vi "SSC DCPower Source Voltage v2.vi"(0 "DCPower SSC in":T1[](array[typedef]), 5 "Voltage Level, V":dbl, 9 "Voltage Level Range (V)":dbl format="%#_6p", 11 "error in":errorcluster, 12 "Current Limit, A":dbl, 14 "Current Limit Range (A)":dbl format="%#_6p") -> (4 "DCPower SSC out":T1[](array[typedef]), 15 "error out":errorcluster)   [LabVIEW 2019]
uses:
  SSC DCPower.ctl
  <instrlib>/niDCPower/nidcpower.llb/niDCPower Output Function.ctl
  <instrlib>/niDCPower/nidcpower.llb/niDCPower Source Mode.ctl
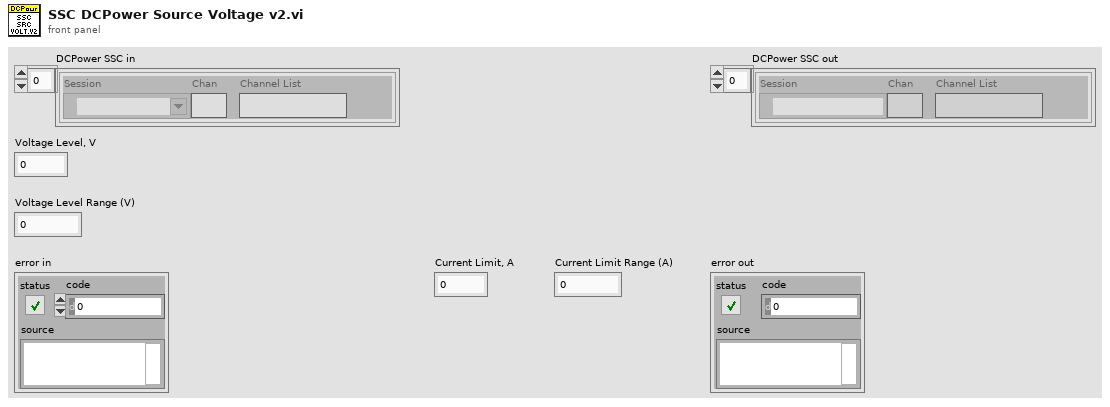
[diagram p1: front panel]
types:
  T1 = typedef "SSC DCPower.ctl" = cluster{"Session":refnum<k15>, "Chan":string, "Channel List":string}
  T2 = typedef "niDCPower Source Mode.ctl" = i32
  T3 = typedef "niDCPower Output Function.ctl" = i32
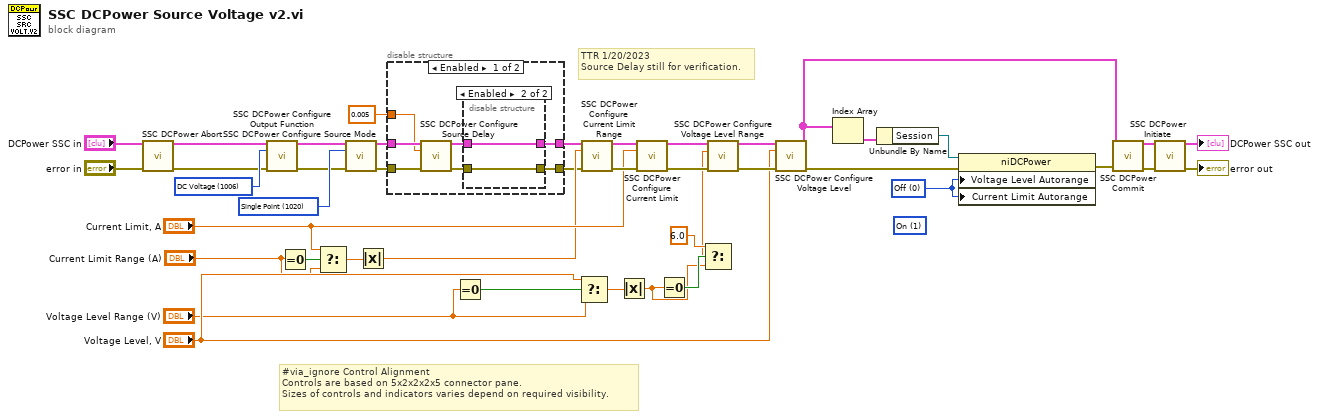
[diagram p0: block diagram]
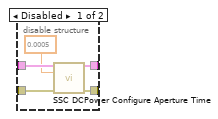
[diagram p2: hidden frame]
diagram:
  (unwired) 1 items=["Off", "On"] ("Source:DC Voltage:Voltage Level Autorange")
  w1 = 0 items=["Off", "On"] ("Source:DC Voltage:Voltage Level Autorange")
  w18 = T2 1020 items=["Single Point"=1020, "Sequence"=1021] ("Source Mode")
  w42 = T3 1006 items=["DC Voltage"=1006, "DC Current"=1007, "Pulse Voltage"=1049, "Pulse Current"=1050] ("Output Function")
  # "TTR 1/20/2023\nSource Delay still for verification."
  # "#via_ignore Control Alignment\nControls are based on 5x2x2x2x5 connector pane.\nSizes of controls and indicators varies depend on required visibility."
  n1 = call "SSC DCPower Abort.vi"("DCPower SSC in"="DCPower SSC in", "error in"="error in") -> ("DCPower SSC out"=w32:T1[], "error out"=w34:errorcluster)  [unwired: 12 in]
  n2 = call "SSC DCPower Configure Output Function.vi"("DCPower SSC in"=w32, "Output Function"=w42, "error in"=w34) -> ("DCPower SSC out"=w17:T1[], "error out"=w16:errorcluster)  [unwired: 11 in]
  n3 = Equal To 0?(x="Current Limit Range (A)") -> (x = 0?=w22:bool)
  n4 = Select(t="Current Limit, A", s=w22, f="Current Limit Range (A)") -> (s? t:f=w23:dbl)
  n5 = call "SSC DCPower Configure Source Mode.vi"("DCPower SSC in"=w17, "Source Mode"=w18, "error in"=w16) -> ("DCPower SSC out"=w11:T1[], "error out"=w9:errorcluster)  [unwired: 11 in]
  n6 = Absolute Value(x=w23) -> (abs(x)=w19:dbl)
  n7 = disable-structure shown="Enabled" {
    disable-tunnel: w11 -> [w49 w58]
    disable-tunnel: [w46 w58] -> w10
    disable-tunnel: w9 -> [w48 w57]
    disable-tunnel: [w44 w57] -> w8
    disable-tunnel: 0.005 ("Source Delay (s)") -> [w43 _]
    frame Enabled {
      n8 = call "SSC DCPower Configure Source Delay.vi"("DCPower SSC in"=w49, "Source Delay (s)"=w43, "error in"=w48) -> ("DCPower SSC out"=w47:T1[], "error out"=w45:errorcluster)  [unwired: 11 in]
      n9 = disable-structure shown="Enabled" {
        disable-tunnel: w47 -> [w54 w56]
        disable-tunnel: [w53 w56] -> w46
        disable-tunnel: w45 -> [w52 w55]
        disable-tunnel: [w51 w55] -> w44
        frame Disabled {
          n10 = call "SSC DCPower Configure Aperture Time.vi"("DCPower SSC in"=w54, "Aperture Time"=0.0005, "error in"=w52) -> ("DCPower SSC out"=w53:T1[], "error out"=w51:errorcluster)  [unwired: 11 in]
        }
        frame Enabled {
        }
      }
    }
    frame Disabled {
    }
  }
  n11 = Equal To 0?(x="Voltage Level Range (V)") -> (x = 0?=w27:bool)
  n12 = Select(t="Voltage Level, V", s=w27, f="Voltage Level Range (V)") -> (s? t:f=w24:dbl)
  n13 = call "SSC DCPower Configure Current Limit Range.vi"("DCPower SSC in"=w10, "Current Limit Range (A)"=w19, "error in"=w8) -> ("DCPower SSC out"=w40:T1[], "error out"=w39:errorcluster)  [unwired: 11 in]
  n14 = Absolute Value(x=w24) -> (abs(x)=w14:dbl)
  n15 = call "SSC DCPower Configure Current Limit.vi"("DCPower SSC in"=w40, "Current Limit (A)"="Current Limit, A", "error in"=w39) -> ("DCPower SSC out"=w38:T1[], "error out"=w37:errorcluster)  [unwired: 11 in]
  n16 = Equal To 0?(x=w14) -> (x = 0?=w15:bool)
  n17 = Select(t=6.0, s=w15, f=w14) -> (s? t:f=w12:dbl)
  n18 = call "SSC DCPower Configure Voltage Level Range.vi"("DCPower SSC in"=w38, "Voltage Level Range (V)"=w12, "error in"=w37) -> ("DCPower SSC out"=w36:T1[], "error out"=w35:errorcluster)  [unwired: 11 in]
  n19 = call "SSC DCPower Configure Voltage Level.vi"("DCPower SSC in"=w36, "Voltage Level (V)"="Voltage Level, V", "error in"=w35) -> ("DCPower SSC out"=w4:T1[], "error out"=w3:errorcluster)  [unwired: 11 in]
  n20 = Index Array(array=w4) -> (element=w6:T1)  [unwired: 1 in]
  n21 = Unbundle By Name(w6) -> ("Session"=w5:refnum<k15>)
  n22 = property class="niDCPower"(reference=w5, error in=w3, "Voltage Level Autorange"=w1, "Current Limit Autorange"=w1) -> (error out=w2:errorcluster)  [unwired: 1 out]
  n23 = call "SSC DCPower Commit.vi"("DCPower SSC in"=w4, "error in"=w2) -> ("DCPower SSC out"=w29:T1[], "error out"=w31:errorcluster)  [unwired: 12 in]
  n24 = call "SSC DCPower Initiate.vi"("DCPower SSC in"=w29, "error in"=w31) -> ("DCPower SSC out"=→"DCPower SSC out":T1[], "error out"=→"error out":errorcluster)  [unwired: 12 in]
